vi "LVCAM Msg Receive.vi"(11 "Process in":refnum<class "ABD.lvclass">) -> (0 "error out":errorcluster, 2 "Msg":refnum<class "Msg.lvclass">)   [LabVIEW 2021, in "ABD.lvlib" / "ABD.lvclass"]
uses:
  ABD.lvclass
  LVCAM/LVCAM/Msg/Msg.lvclass
  ABD.lvclass/ABD.ctl
  LVCAM/LVCAM/LVCAM/LVCAM.lvclass
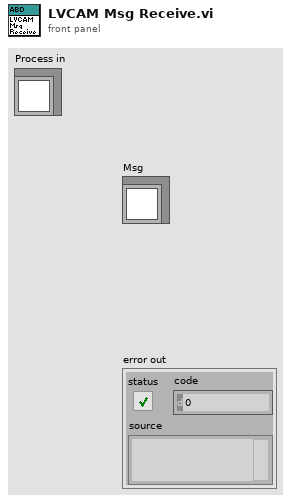
[diagram p1: front panel]
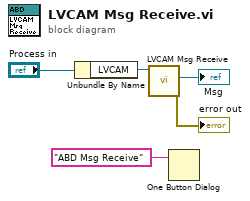
[diagram p0: block diagram]
diagram:
  n1 = Unbundle By Name("Process in") -> ("LVCAM"=w2:refnum<class "LVCAM.lvclass">)
  n2 = call-dynamic "LVCAM Msg Receive.vi"("LVCAM Msg Receive in"=w2) -> ("error out"=→"error out":errorcluster, "Msg"=→"Msg":refnum<class "Msg.lvclass">)  [unwired: 9 in]
  n3 = One Button Dialog(message="ABD Msg Receive") -> ()  [unwired: 1 in, 1 out]
